vi "Create All Message Queues.vi"(8 "error in (no error)":errorcluster) -> (0 "error out":errorcluster, 3 "Message Queues Out":T1)   [LabVIEW 2014, in "Message Queue.lvlib"]
doc: "This VI creates and initializes all the message queues for your application. If your application requires more than one message queue, right-click the \"Message Queues\" constant above and select Open Type Def. Add the new Message Queue(s) to the type definition, then initialize them in this VI."
uses:
  Message Queue.lvlib
  All Message Queues.ctl
  Message Cluster.ctl
  Enqueue Message (Single).vi
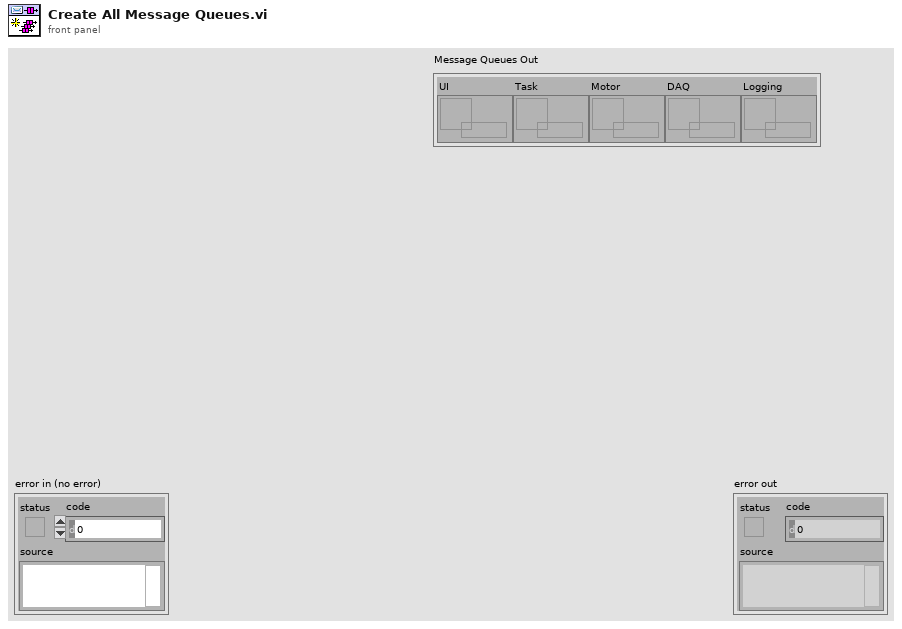
[diagram p1: front panel]
types:
  T1 = typedef "Message Queue.lvlib/All Message Queues.ctl" = cluster{"UI":refnum<queue>, "Task":refnum<queue>, "Motor":refnum<queue>, "DAQ":refnum<queue>, "Logging":refnum<queue>}
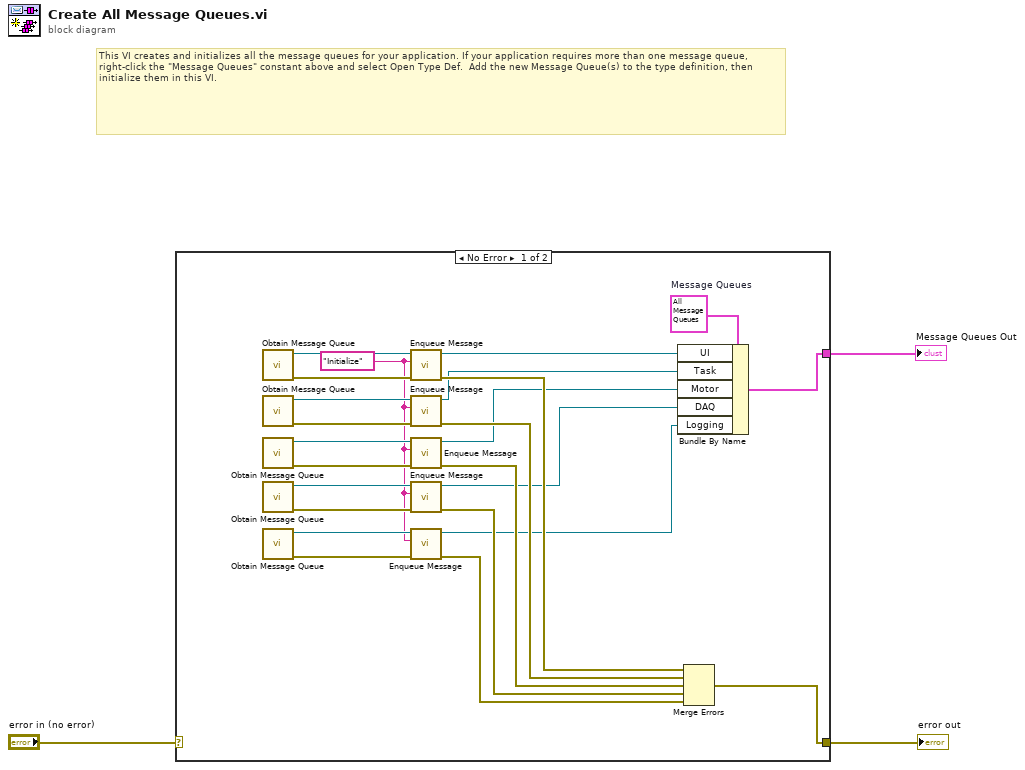
[diagram p0: block diagram]
diagram:
  # "This VI creates and initializes all the message queues for your application. If your application requires more than one message queue, right-click the \"Message Queues\" constant above and select Open Type Def.  Add the new Message Queue(s) to the type definition, then initialize them in this VI."
  n1 = case shown="No Error" "error in (no error)" {
    selector: "error in (no error)" -> [_ w28]
    tunnel: [w9 w28] -> w3
    tunnel: [w26 _] -> w2
    frame No Error {
      w8 = "Initialize" ("Message")
      w27 = T1 {"UI"=refnum, "Task"=refnum, "Motor"=refnum, "DAQ"=refnum, "Logging"=refnum}  # Message Queues
      n2 = call "Obtain Message Queue.vi"() -> ("error out"=w25:errorcluster, "Message Queue"=w24:refnum<queue>)  [unwired: 10 in]
      n3 = call "Obtain Message Queue.vi"() -> ("error out"=w19:errorcluster, "Message Queue"=w20:refnum<queue>)  [unwired: 10 in]
      n4 = call "Obtain Message Queue.vi"() -> ("error out"=w17:errorcluster, "Message Queue"=w18:refnum<queue>)  [unwired: 10 in]
      n5 = call "Obtain Message Queue.vi"() -> ("error out"=w15:errorcluster, "Message Queue"=w16:refnum<queue>)  [unwired: 10 in]
      n6 = call "Obtain Message Queue.vi"() -> ("error out"=w21:errorcluster, "Message Queue"=w22:refnum<queue>)  [unwired: 10 in]
      n7 = call-poly "Enqueue Message.vi"("error in (no error)"=w25, "Message"=w8, "Message Queue"=w24) -> ("error out"=w14:errorcluster, "dup Message Queue"=w23:refnum<queue>)  [unwired: 7 in]
      n8 = call-poly "Enqueue Message.vi"("error in (no error)"=w19, "Message"=w8, "Message Queue"=w20) -> ("error out"=w10:errorcluster, "dup Message Queue"=w7:refnum<queue>)  [unwired: 7 in]
      n9 = call-poly "Enqueue Message.vi"("error in (no error)"=w17, "Message"=w8, "Message Queue"=w18) -> ("error out"=w11:errorcluster, "dup Message Queue"=w4:refnum<queue>)  [unwired: 7 in]
      n10 = call-poly "Enqueue Message.vi"("error in (no error)"=w15, "Message"=w8, "Message Queue"=w16) -> ("error out"=w12:errorcluster, "dup Message Queue"=w5:refnum<queue>)  [unwired: 7 in]
      n11 = call-poly "Enqueue Message.vi"("error in (no error)"=w21, "Message"=w8, "Message Queue"=w22) -> ("error out"=w13:errorcluster, "dup Message Queue"=w6:refnum<queue>)  [unwired: 7 in]
      n12 = Bundle By Name(cluster=w27, "UI"=w23, "Task"=w7, "Motor"=w4, "DAQ"=w5, "Logging"=w6) -> (w26:T1)
      n13 = Merge Errors(w14, w10, w11, w12, w13) -> (w9:errorcluster)
    }
    frame Error {
    }
  }
  "Message Queues Out" <- w2
  "error out" <- w3
